vi "tool_Unicode_Convert Unicode to ASCII (2D).vi"(4 "Unicode":string[][](array[string])) -> (1 "ASCII":string[][](array[string]))   [LabVIEW 2009]
uses:
  kernel32.dll
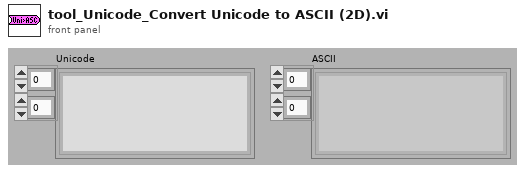
[diagram p1: front panel]
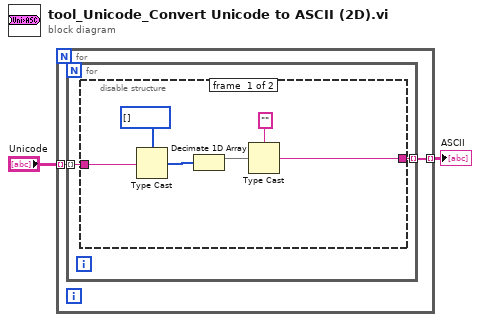
[diagram p0: block diagram]
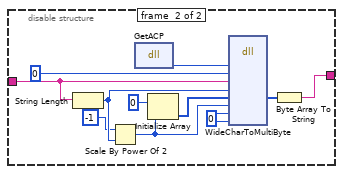
[diagram p2: hidden frame]
diagram:
  n1 = for {
    tunnel: "Unicode" -> [w4] mode=indexing
    tunnel: [w3] -> w1 mode=indexing
    n2 = for {
      tunnel: w4 -> [w6] mode=indexing
      tunnel: [w5] -> w3 mode=indexing
      n3 = disable-structure shown="Enabled" {
        disable-tunnel: w6 -> [w12 w18]
        disable-tunnel: [w9 w17] -> w5
        frame #0 {
          n4 = Type Cast(type=u8[] [], x=w12) -> (*(type *) &x=w8:u8[])
          n5 = Decimate 1D Array(w8) -> (w7:u8[])  [unwired: 1 out]
          n6 = Type Cast(type="", x=w7) -> (*(type *) &x=w9:string)
        }
        frame #1 {
          w13 = u32 0
          n7 = String Length(string=w18) -> (length=w16:i32)
          n8 = Scale By Power Of 2(n=-1, x=w16) -> (x*2^n=w14:i32)
          n9 = dll-call lib="kernel32.dll" fn="GetACP" label="GetACP()"() -> (w23:u32)  [unwired: 3 in, 2 out]
          n10 = Initialize Array(u8 0, w14) -> (w21:u8[])
          n11 = dll-call lib="kernel32.dll" fn="WideCharToMultiByte"("codePage"=w23, "dwFlags"=u32 0, "lpWideCharStr"=w18, "cchWideChar"=w16, "lpMultiByteStr"=w21, "cbMultiByte"=w14, "lpDefaultChar"=w13, "lpUsedDefaultChar"=w13) -> ("lpMultiByteStr"=w22:u8[])  [unwired: 10 in, 3 out]
          n12 = Byte Array To String(unsigned byte array=w22) -> (string=w17:string)
        }
      }
    }
  }
  "ASCII" <- w1
